vi "fpga_main.vi"() -> ()   [LabVIEW 2023]
panel:
  out "ANALOG_OUTPUT_VALUE":i16
  in  "VALUE":i16
  in  "ANALOG_DIGITAL_SELECTOR":bool
  in  "PIN_MODE":bool
  in  "PIN_MODE_EN":bool
  in  "VALUE":bool
  out "DIGITAL_OUTPUT_VALUE":bool
  in  "ENABLE":bool
  in  "PIN":u16
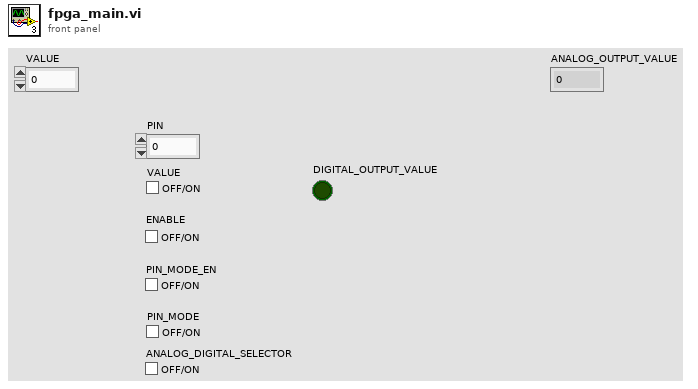
[diagram p1: front panel]
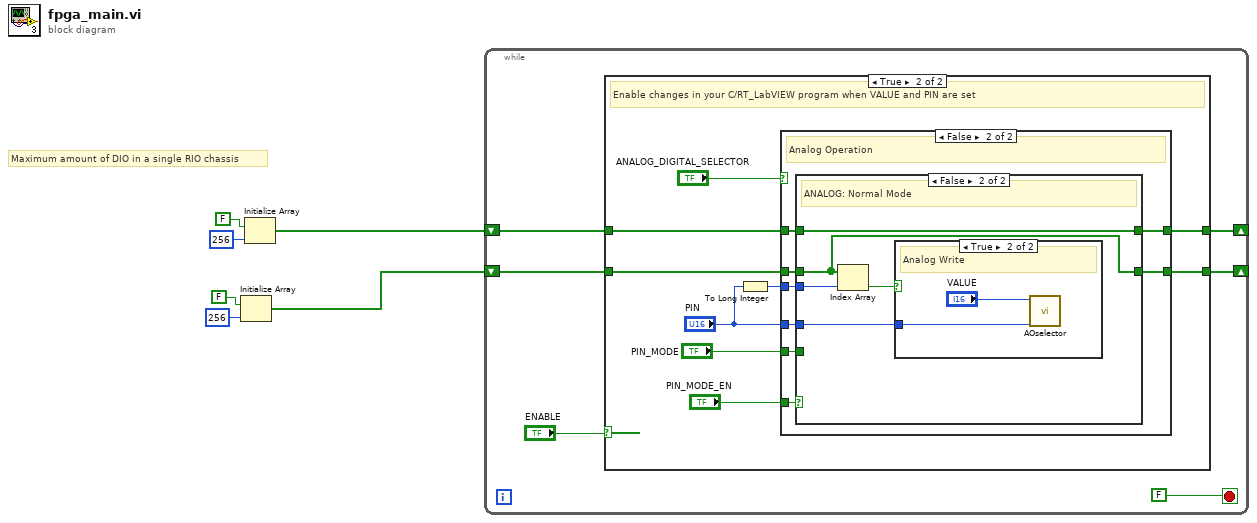
[diagram p0: block diagram]
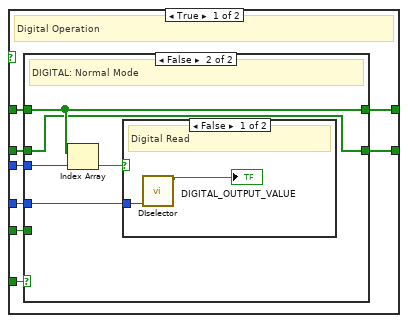
[diagram p3: hidden frame]
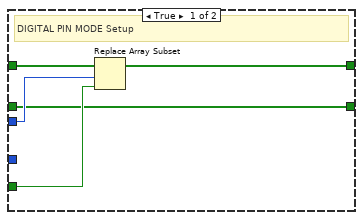
[diagram p4: hidden frame]
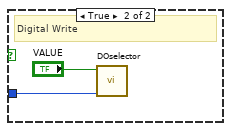
[diagram p5: hidden frame]
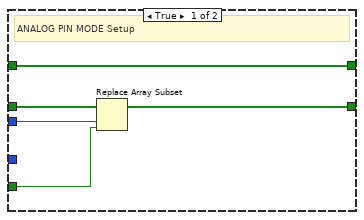
[diagram p6: hidden frame]
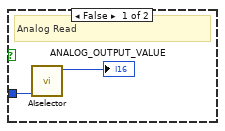
[diagram p7: hidden frame]
diagram:
  # "Maximum amount of DIO in a single RIO chassis"
  n1 = Initialize Array(FALSE, 256 ("dimension size")) -> (w1:bool[])
  n2 = Initialize Array(FALSE, 256 ("dimension size")) -> (w4:bool[])
  n3 = while {
    shift-right: [w9] -> _
    shift-left: w4 -> [w11]
    shift-right: [w7] -> _
    shift-left: w1 -> [w8]
    stop <- FALSE stop-if-true
    n4 = case shown="True" "ENABLE" {
      tunnel: w11 -> [w14 w23]
      tunnel: [w14 w20] -> w9
      tunnel: w8 -> [w13 w17]
      tunnel: [w13 w16] -> w7
      frame False {
      }
      frame True {
        # "Enable changes in your C/RT_LabVIEW program when VALUE and PIN are set"
        n5 = To Long Integer(number="PIN") -> (32bit integer=w22:i32)
        n6 = case shown="False" "ANALOG_DIGITAL_SELECTOR" {
          tunnel: w23 -> [w31 w50]
          tunnel: w22 -> [w30 w53]
          tunnel: "PIN" -> [w29 w52]
          tunnel: [w28 w49] -> w20
          tunnel: "PIN_MODE_EN" -> [w27 w51]
          tunnel: w17 -> [w25 w48]
          tunnel: [w24 w47] -> w16
          tunnel: "PIN_MODE" -> [w26 w46]
          frame True {
            # "Digital Operation"
            n7 = case shown="False" w27 {
              tunnel: w31 -> [w36 w38]
              tunnel: w30 -> [w34 w40]
              tunnel: w29 -> [_ w39]
              tunnel: [w35 w38] -> w28
              tunnel: w26 -> [w33 _]
              tunnel: w25 -> [w32 w37]
              tunnel: [w32 w37] -> w24
              frame True {
                # "DIGITAL PIN MODE Setup"
                n8 = Replace Array Subset(array=w36, new element=w33, index=w34) -> (w35:bool[])
              }
              frame False {
                # "DIGITAL: Normal Mode"
                n9 = Index Array(array=w38, index=w40) -> (element=w41:bool)
                n10 = case shown="False" w41 {
                  tunnel: w39 -> [w42 w45]
                  frame False {
                    # "Digital Read"
                    n11 = call "DIselector.vi"("I/O element"=w42) -> ("value"=→"DIGITAL_OUTPUT_VALUE":bool)  [unwired: 10 in]
                  }
                  frame True {
                    # "Digital Write"
                    n12 = call "DOselector.vi"("I/O element"=w45, "value"="VALUE") -> ()  [unwired: 10 in]
                  }
                }
              }
            }
          }
          frame False {
            # "Analog Operation"
            n13 = case shown="False" w51 {
              tunnel: w53 -> [w58 w63]
              tunnel: w52 -> [_ w62]
              tunnel: w50 -> [w57 w61]
              tunnel: [w57 w61] -> w49
              tunnel: w48 -> [w56 w59]
              tunnel: [w55 w59] -> w47
              tunnel: w46 -> [w54 _]
              frame True {
                # "ANALOG PIN MODE Setup"
                n14 = Replace Array Subset(array=w56, new element=w54, index=w58) -> (w55:bool[])
              }
              frame False {
                # "ANALOG: Normal Mode"
                n15 = Index Array(array=w59, index=w63) -> (element=w60:bool)
                n16 = case shown="True" w60 {
                  tunnel: w62 -> [w65 w67]
                  frame False {
                    # "Analog Read"
                    n17 = call "AIselector.vi"("I/O element"=w65) -> ("value"=→"ANALOG_OUTPUT_VALUE":i16)  [unwired: 10 in]
                  }
                  frame True {
                    # "Analog Write"
                    n18 = call "AOselector.vi"("I/O element"=w67, "value"="VALUE") -> ()  [unwired: 10 in]
                  }
                }
              }
            }
          }
        }
      }
    }
  }
